vi "Finish.vi"   [LabVIEW 2019]
doc: "This VI is called just before exiting. It is expected to close I/O refnum, save collected data, etc."
uses:
  refnums.vi
  <vilib>/Rock Robotics/WPI/Utilities/WPI_GetSetVariantRefNum.vi
types:
  T1 = typedef "WPI_MotorControlDeviceRef.ctl" = cluster{"DeviceStatus":errorcluster, "Type":T2, "PWM":cluster{"PWM Channel":T3, "DeadBand":T4}, "CAN":cluster{"Device Number":u8, "SetOutput VI Ref":variant, "GetOutput VI Ref":variant, "Enable VI Ref":variant, "Disable VI Ref":variant, "Data":variant}, "Invert":bool, "DIO PWM":cluster{"PWM \"Enable\" Channel":T3, "DIOChannel":T5, "PWM Rate":dbl}}
  T2 = typedef "WPI_MotorControlType.ctl" = enum16{"PWM", "CAN", "DIO PWM"}
  T3 = typedef "FPGA_DIOPWMChannel.ctl" = enum8{"PWM 0", "PWM 1", "PWM 2", "PWM 3", "PWM 4", "PWM 5", "PWM 6", "PWM 7", "PWM 8", "PWM 9", "PWM MXP 0", "PWM MXP 1", "PWM MXP 2", "PWM MXP 3", "PWM MXP 4", "PWM MXP 5", "PWM MXP 6", "PWM MXP 7", "PWM MXP 8", "PWM MXP 9", "Invalid"}
  T4 = typedef "WPI_PWMDeadband.ctl" = cluster{"Name":string, "maxPositivePwm":i32, "minPositivePwm":i32, "centerPwm":i32, "maxNegativePwm":i32, "minNegativePwm":i32, "angularRange":u16}
  T5 = typedef "FPGA_DIOChannel.ctl" = enum8{"DIO 0", "DIO 1", "DIO 2", "DIO 3", "DIO 4", "DIO 5", "DIO 6", "DIO 7", "DIO 8", "DIO 9", "DIO MXP 0", "DIO MXP 1", "DIO MXP 2", "DIO MXP 3", "DIO MXP 4", "DIO MXP 5", "DIO MXP 6", "DIO MXP 7", "DIO MXP 8", "DIO MXP 9", "DIO MXP 10", "DIO MXP 11", "DIO MXP 12", "DIO MXP 13", "DIO MXP 14", "DIO MXP 15", "SPI Port CS1", "SPI Port CS2", "SPI Port CS3", "SPI Port MISO", "SPI Port MOSI", "Invalid"}
  T6 = typedef "WPI_PotentiometerDevRef.ctl" = cluster{"DevStatus":errorcluster, "Analog Channel":T7, "Invert Output":bool}
  T7 = typedef "FPGA_AIChannel.ctl" = enum8{"AI 0", "AI 1", "AI 2", "AI 3", "AI MXP 0", "AI MXP 1", "AI MXP 2", "AI MXP 3", "Invalid"}
  T8 = typedef "WPI_AnalogChannelDevRef.ctl" = cluster{"DevStatus":errorcluster, "Analog Channel":T7}
  T9 = typedef "WPI_SolenoidDevRef.ctl" = cluster{"DevStatus":errorcluster, "Pneumatics Control Module":u8, "Forward Solenoid Channel":T10, "Reverse Solenoid Channel":T10}
  T10 = typedef "WPI_SolenoidChannel.ctl" = enum8{"Solenoid 0", "Solenoid 1", "Solenoid 2", "Solenoid 3", "Solenoid 4", "Solenoid 5", "Solenoid 6", "Solenoid 7", "Invalid"}
  T11 = typedef "WPI_SwitchDevRef.ctl" = cluster{"DevStatus":errorcluster, "DIO Channel":T5, "CntIndex":T12, "Normally Closed":bool}
  T12 = typedef "FPGA_CounterCtrSystemIndex.ctl" = enum8{"Ctr 0", "Ctr 1", "Ctr 2", "Ctr 3", "Ctr 4", "Ctr 5", "Ctr 6", "Ctr 7", "Invalid"}
  T13 = typedef "WPI_CounterDevRef.ctl" = cluster{"DevStatus":errorcluster, "CntIndex":T12}
  T14 = typedef "WPI_JoystickDevRef.ctl" = cluster{"Device":T15}
  T15 = typedef "WPI_JoystickDeviceEnum.ctl" = enum16{"USB 0", "USB 1", "USB 2", "USB 3", "USB 4", "USB 5"}
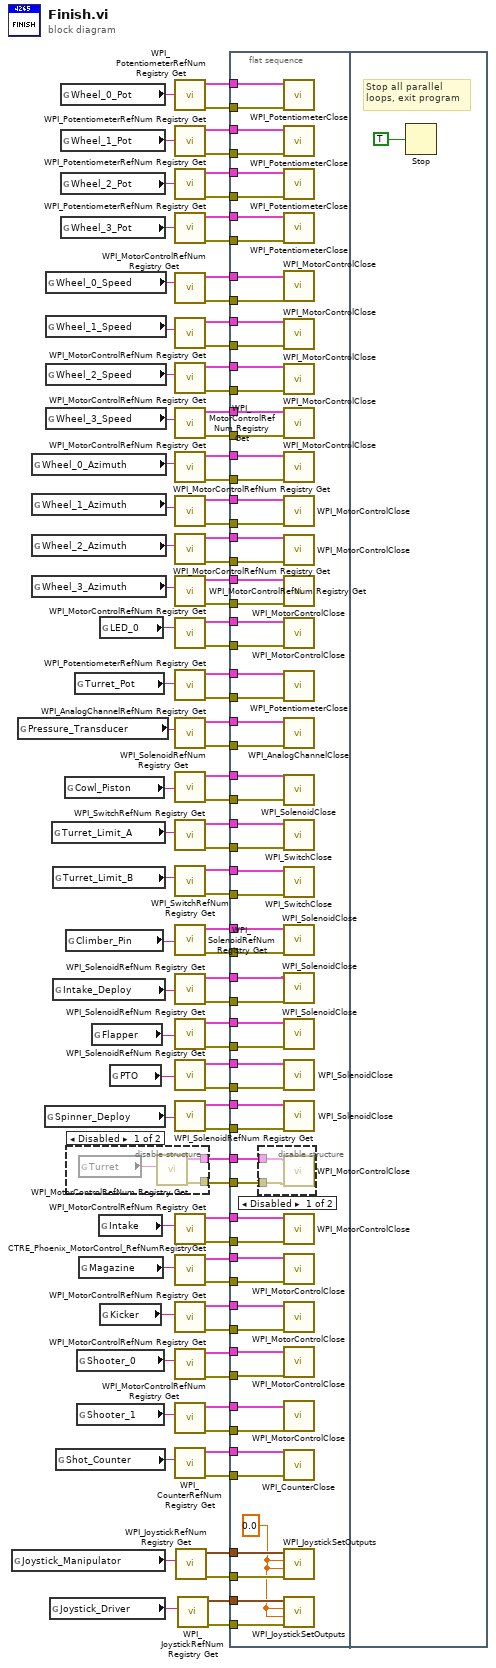
[diagram p0: block diagram]
diagram:
  n1 = global read "refnums.vi" "Joystick_Manipulator"() -> (w6:string)
  n2 = global read "refnums.vi" "Pressure_Transducer"() -> (w56:string)
  n3 = global read "refnums.vi" "Wheel_0_Azimuth"() -> (w83:string)
  n4 = global read "refnums.vi" "Wheel_1_Azimuth"() -> (w82:string)
  n5 = global read "refnums.vi" "Wheel_2_Azimuth"() -> (w81:string)
  n6 = global read "refnums.vi" "Wheel_3_Azimuth"() -> (w80:string)
  n7 = global read "refnums.vi" "Spinner_Deploy"() -> (w21:string)
  n8 = global read "refnums.vi" "Wheel_0_Speed"() -> (w87:string)
  n9 = global read "refnums.vi" "Wheel_1_Speed"() -> (w86:string)
  n10 = global read "refnums.vi" "Wheel_2_Speed"() -> (w85:string)
  n11 = global read "refnums.vi" "Wheel_3_Speed"() -> (w84:string)
  n12 = global read "refnums.vi" "Joystick_Driver"() -> (w1:string)
  n13 = global read "refnums.vi" "Turret_Limit_A"() -> (w11:string)
  n14 = global read "refnums.vi" "Turret_Limit_B"() -> (w10:string)
  n15 = global read "refnums.vi" "Intake_Deploy"() -> (w30:string)
  n16 = global read "refnums.vi" "Shot_Counter"() -> (w8:string)
  n17 = global read "refnums.vi" "Wheel_0_Pot"() -> (w95:string)
  n18 = global read "refnums.vi" "Wheel_1_Pot"() -> (w93:string)
  n19 = global read "refnums.vi" "Wheel_2_Pot"() -> (w92:string)
  n20 = global read "refnums.vi" "Wheel_3_Pot"() -> (w91:string)
  n21 = global read "refnums.vi" "Cowl_Piston"() -> (w53:string)
  n22 = global read "refnums.vi" "Climber_Pin"() -> (w33:string)
  n23 = disable-structure shown="Disabled" {
    disable-tunnel: [w97 _] -> w35
    disable-tunnel: [w96 _] -> w34
    frame Disabled {
      n24 = global read "refnums.vi" "Turret"() -> (w98:string)
      n25 = call <vilib>:"WPI_MotorControlRefNum Registry Get.vi"("refnum name"=w98) -> ("error out"=w96:errorcluster, "MotorControlDevRef"=w97:T1)  [unwired: 9 in]
    }
    frame Enabled {
    }
  }
  n26 = global read "refnums.vi" "Turret_Pot"() -> (w18:string)
  n27 = global read "refnums.vi" "Shooter_0"() -> (w45:string)
  n28 = global read "refnums.vi" "Shooter_1"() -> (w44:string)
  n29 = global read "refnums.vi" "Magazine"() -> (w50:string)
  n30 = global read "refnums.vi" "Flapper"() -> (w29:string)
  n31 = global read "refnums.vi" "Intake"() -> (w38:string)
  n32 = global read "refnums.vi" "LED_0"() -> (w71:string)
  n33 = global read "refnums.vi" "Kicker"() -> (w41:string)
  n34 = global read "refnums.vi" "PTO"() -> (w24:string)
  n35 = call <vilib>:"WPI_PotentiometerRefNum Registry Get.vi"("refnum name"=w95) -> ("error out"=w69:errorcluster, "PotDevRef"=w94:T6)  [unwired: 9 in]
  n36 = call <vilib>:"WPI_PotentiometerRefNum Registry Get.vi"("refnum name"=w93) -> ("error out"=w68:errorcluster, "PotDevRef"=w90:T6)  [unwired: 9 in]
  n37 = call <vilib>:"WPI_PotentiometerRefNum Registry Get.vi"("refnum name"=w92) -> ("error out"=w67:errorcluster, "PotDevRef"=w89:T6)  [unwired: 9 in]
  n38 = call <vilib>:"WPI_PotentiometerRefNum Registry Get.vi"("refnum name"=w91) -> ("error out"=w66:errorcluster, "PotDevRef"=w88:T6)  [unwired: 9 in]
  n39 = call <vilib>:"WPI_MotorControlRefNum Registry Get.vi"("refnum name"=w87) -> ("error out"=w65:errorcluster, "MotorControlDevRef"=w79:T1)  [unwired: 9 in]
  n40 = call <vilib>:"WPI_MotorControlRefNum Registry Get.vi"("refnum name"=w86) -> ("error out"=w64:errorcluster, "MotorControlDevRef"=w78:T1)  [unwired: 9 in]
  n41 = call <vilib>:"WPI_MotorControlRefNum Registry Get.vi"("refnum name"=w85) -> ("error out"=w63:errorcluster, "MotorControlDevRef"=w77:T1)  [unwired: 9 in]
  n42 = call <vilib>:"WPI_MotorControlRefNum Registry Get.vi"("refnum name"=w84) -> ("error out"=w62:errorcluster, "MotorControlDevRef"=w76:T1)  [unwired: 9 in]
  n43 = call <vilib>:"WPI_MotorControlRefNum Registry Get.vi"("refnum name"=w83) -> ("error out"=w61:errorcluster, "MotorControlDevRef"=w75:T1)  [unwired: 9 in]
  n44 = call <vilib>:"WPI_MotorControlRefNum Registry Get.vi"("refnum name"=w82) -> ("error out"=w60:errorcluster, "MotorControlDevRef"=w74:T1)  [unwired: 9 in]
  n45 = call <vilib>:"WPI_MotorControlRefNum Registry Get.vi"("refnum name"=w81) -> ("error out"=w59:errorcluster, "MotorControlDevRef"=w73:T1)  [unwired: 9 in]
  n46 = call <vilib>:"WPI_MotorControlRefNum Registry Get.vi"("refnum name"=w80) -> ("error out"=w58:errorcluster, "MotorControlDevRef"=w72:T1)  [unwired: 9 in]
  n47 = call <vilib>:"WPI_MotorControlRefNum Registry Get.vi"("refnum name"=w71) -> ("error out"=w57:errorcluster, "MotorControlDevRef"=w70:T1)  [unwired: 9 in]
  n48 = call <vilib>:"WPI_PotentiometerRefNum Registry Get.vi"("refnum name"=w18) -> ("error out"=w16:errorcluster, "PotDevRef"=w17:T6)  [unwired: 9 in]
  n49 = call <vilib>:"WPI_AnalogChannelRefNum Registry Get.vi"("refnum name"=w56) -> ("error out"=w54:errorcluster, "AIDeviceRef"=w55:T8)  [unwired: 9 in]
  n50 = call <vilib>:"WPI_SolenoidRefNum Registry Get.vi"("refnum name"=w53) -> ("error out"=w51:errorcluster, "SolenoidDevRef"=w52:T9)  [unwired: 9 in]
  n51 = call <vilib>:"WPI_SwitchRefNum Registry Get.vi"("refnum name"=w11) -> ("error out"=w14:errorcluster, "SwitchDevRef"=w15:T11)  [unwired: 9 in]
  n52 = call <vilib>:"WPI_SwitchRefNum Registry Get.vi"("refnum name"=w10) -> ("error out"=w12:errorcluster, "SwitchDevRef"=w13:T11)  [unwired: 9 in]
  n53 = call <vilib>:"WPI_SolenoidRefNum Registry Get.vi"("refnum name"=w33) -> ("error out"=w31:errorcluster, "SolenoidDevRef"=w32:T9)  [unwired: 9 in]
  n54 = call <vilib>:"WPI_SolenoidRefNum Registry Get.vi"("refnum name"=w30) -> ("error out"=w27:errorcluster, "SolenoidDevRef"=w28:T9)  [unwired: 9 in]
  n55 = call <vilib>:"WPI_SolenoidRefNum Registry Get.vi"("refnum name"=w29) -> ("error out"=w25:errorcluster, "SolenoidDevRef"=w26:T9)  [unwired: 9 in]
  n56 = call <vilib>:"WPI_SolenoidRefNum Registry Get.vi"("refnum name"=w24) -> ("error out"=w22:errorcluster, "SolenoidDevRef"=w23:T9)  [unwired: 9 in]
  n57 = call <vilib>:"WPI_SolenoidRefNum Registry Get.vi"("refnum name"=w21) -> ("error out"=w19:errorcluster, "SolenoidDevRef"=w20:T9)  [unwired: 9 in]
  n58 = call <vilib>:"WPI_MotorControlRefNum Registry Get.vi"("refnum name"=w38) -> ("error out"=w36:errorcluster, "MotorControlDevRef"=w37:T1)  [unwired: 9 in]
  n59 = call <vilib>:"CTRE_Phoenix_MotorControl_RefNumRegistryGet.vi"("refnum name"=w50) -> ("error out"=w48:errorcluster, "PhoenixMotorControlDevRef"=w49:T1)  [unwired: 9 in]
  n60 = call <vilib>:"WPI_MotorControlRefNum Registry Get.vi"("refnum name"=w41) -> ("error out"=w39:errorcluster, "MotorControlDevRef"=w40:T1)  [unwired: 9 in]
  n61 = call <vilib>:"WPI_MotorControlRefNum Registry Get.vi"("refnum name"=w45) -> ("error out"=w46:errorcluster, "MotorControlDevRef"=w47:T1)  [unwired: 9 in]
  n62 = call <vilib>:"WPI_MotorControlRefNum Registry Get.vi"("refnum name"=w44) -> ("error out"=w42:errorcluster, "MotorControlDevRef"=w43:T1)  [unwired: 9 in]
  n63 = call <vilib>:"WPI_CounterRefNum Registry Get.vi"("refnum name"=w8) -> ("error out"=w7:errorcluster, "CounterDevRef"=w9:T13)  [unwired: 9 in]
  n64 = call <vilib>:"WPI_JoystickRefNum Registry Get.vi"("refnum name"=w6) -> ("error out"=w4:errorcluster, "JoystickDevRef"=w5:T14)  [unwired: 9 in]
  n65 = call <vilib>:"WPI_JoystickRefNum Registry Get.vi"("refnum name"=w1) -> ("error out"=w2:errorcluster, "JoystickDevRef"=w3:T14)  [unwired: 9 in]
  n66 = flat-sequence {
    tunnel: w94 -> [w163]
    tunnel: w90 -> [w162]
    tunnel: w89 -> [w161]
    tunnel: w88 -> [w160]
    tunnel: w79 -> [w159]
    tunnel: w78 -> [w158]
    tunnel: w77 -> [w157]
    tunnel: w76 -> [w156]
    tunnel: w75 -> [w155]
    tunnel: w74 -> [w154]
    tunnel: w73 -> [w153]
    tunnel: w72 -> [w152]
    tunnel: w70 -> [w151]
    tunnel: w69 -> [w150]
    tunnel: w68 -> [w149]
    tunnel: w67 -> [w148]
    tunnel: w66 -> [w147]
    tunnel: w65 -> [w146]
    tunnel: w64 -> [w145]
    tunnel: w63 -> [w144]
    tunnel: w62 -> [w143]
    tunnel: w61 -> [w142]
    tunnel: w60 -> [w141]
    tunnel: w59 -> [w140]
    tunnel: w58 -> [w139]
    tunnel: w57 -> [w138]
    tunnel: w55 -> [w137]
    tunnel: w54 -> [w136]
    tunnel: w52 -> [w135]
    tunnel: w51 -> [w134]
    tunnel: w47 -> [w133]
    tunnel: w46 -> [w132]
    tunnel: w49 -> [w131]
    tunnel: w48 -> [w130]
    tunnel: w43 -> [w129]
    tunnel: w42 -> [w128]
    tunnel: w40 -> [w127]
    tunnel: w39 -> [w126]
    tunnel: w37 -> [w125]
    tunnel: w36 -> [w124]
    tunnel: w35 -> [w123]
    tunnel: w34 -> [w122]
    tunnel: w32 -> [w121]
    tunnel: w31 -> [w120]
    tunnel: w28 -> [w119]
    tunnel: w27 -> [w118]
    tunnel: w26 -> [w117]
    tunnel: w25 -> [w116]
    tunnel: w23 -> [w115]
    tunnel: w22 -> [w114]
    tunnel: w20 -> [w113]
    tunnel: w19 -> [w112]
    tunnel: w17 -> [w111]
    tunnel: w16 -> [w110]
    tunnel: w15 -> [w109]
    tunnel: w13 -> [w108]
    tunnel: w12 -> [w107]
    tunnel: w14 -> [w106]
    tunnel: w9 -> [w105]
    tunnel: w7 -> [w104]
    tunnel: w5 -> [w103]
    tunnel: w4 -> [w102]
    tunnel: w3 -> [w101]
    tunnel: w2 -> [w100]
    frame #0 {
      w99 = sgl 0.0 ("Left Rumble")
      n67 = disable-structure shown="Disabled" {
        disable-tunnel: w123 -> [w165 _]
        disable-tunnel: w122 -> [w164 _]
        frame Disabled {
          n68 = call <vilib>:"WPI_MotorControlClose.vi"("error in"=w164, "MotorControlDevRef"=w165) -> ()  [unwired: 9 in, 1 out]
        }
        frame Enabled {
        }
      }
      n69 = call <vilib>:"WPI_PotentiometerClose.vi"("error in"=w150, "PotDevRef"=w163) -> ()  [unwired: 9 in, 1 out]
      n70 = call <vilib>:"WPI_PotentiometerClose.vi"("error in"=w149, "PotDevRef"=w162) -> ()  [unwired: 9 in, 1 out]
      n71 = call <vilib>:"WPI_PotentiometerClose.vi"("error in"=w148, "PotDevRef"=w161) -> ()  [unwired: 9 in, 1 out]
      n72 = call <vilib>:"WPI_PotentiometerClose.vi"("error in"=w147, "PotDevRef"=w160) -> ()  [unwired: 9 in, 1 out]
      n73 = call <vilib>:"WPI_MotorControlClose.vi"("error in"=w146, "MotorControlDevRef"=w159) -> ()  [unwired: 9 in, 1 out]
      n74 = call <vilib>:"WPI_MotorControlClose.vi"("error in"=w145, "MotorControlDevRef"=w158) -> ()  [unwired: 9 in, 1 out]
      n75 = call <vilib>:"WPI_MotorControlClose.vi"("error in"=w144, "MotorControlDevRef"=w157) -> ()  [unwired: 9 in, 1 out]
      n76 = call <vilib>:"WPI_MotorControlClose.vi"("error in"=w143, "MotorControlDevRef"=w156) -> ()  [unwired: 9 in, 1 out]
      n77 = call <vilib>:"WPI_MotorControlClose.vi"("error in"=w142, "MotorControlDevRef"=w155) -> ()  [unwired: 9 in, 1 out]
      n78 = call <vilib>:"WPI_MotorControlClose.vi"("error in"=w141, "MotorControlDevRef"=w154) -> ()  [unwired: 9 in, 1 out]
      n79 = call <vilib>:"WPI_MotorControlClose.vi"("error in"=w140, "MotorControlDevRef"=w153) -> ()  [unwired: 9 in, 1 out]
      n80 = call <vilib>:"WPI_MotorControlClose.vi"("error in"=w139, "MotorControlDevRef"=w152) -> ()  [unwired: 9 in, 1 out]
      n81 = call <vilib>:"WPI_MotorControlClose.vi"("error in"=w138, "MotorControlDevRef"=w151) -> ()  [unwired: 9 in, 1 out]
      n82 = call <vilib>:"WPI_PotentiometerClose.vi"("error in"=w110, "PotDevRef"=w111) -> ()  [unwired: 9 in, 1 out]
      n83 = call <vilib>:"WPI_AnalogChannelClose.vi"("error in (no error)"=w136, "AIDeviceRef"=w137) -> ()  [unwired: 9 in, 1 out]
      n84 = call <vilib>:"WPI_SolenoidClose.vi"("error in (no error)"=w134, "SolenoidDevRef"=w135) -> ()  [unwired: 9 in, 1 out]
      n85 = call <vilib>:"WPI_SwitchClose.vi"("error in (no error)"=w106, "SwitchDevRef"=w109) -> ()  [unwired: 9 in, 1 out]
      n86 = call <vilib>:"WPI_SwitchClose.vi"("error in (no error)"=w107, "SwitchDevRef"=w108) -> ()  [unwired: 9 in, 1 out]
      n87 = call <vilib>:"WPI_SolenoidClose.vi"("error in (no error)"=w120, "SolenoidDevRef"=w121) -> ()  [unwired: 9 in, 1 out]
      n88 = call <vilib>:"WPI_SolenoidClose.vi"("error in (no error)"=w118, "SolenoidDevRef"=w119) -> ()  [unwired: 9 in, 1 out]
      n89 = call <vilib>:"WPI_SolenoidClose.vi"("error in (no error)"=w116, "SolenoidDevRef"=w117) -> ()  [unwired: 9 in, 1 out]
      n90 = call <vilib>:"WPI_SolenoidClose.vi"("error in (no error)"=w114, "SolenoidDevRef"=w115) -> ()  [unwired: 9 in, 1 out]
      n91 = call <vilib>:"WPI_SolenoidClose.vi"("error in (no error)"=w112, "SolenoidDevRef"=w113) -> ()  [unwired: 9 in, 1 out]
      n92 = call <vilib>:"WPI_MotorControlClose.vi"("error in"=w124, "MotorControlDevRef"=w125) -> ()  [unwired: 9 in, 1 out]
      n93 = call <vilib>:"WPI_MotorControlClose.vi"("error in"=w130, "MotorControlDevRef"=w131) -> ()  [unwired: 9 in, 1 out]
      n94 = call <vilib>:"WPI_MotorControlClose.vi"("error in"=w126, "MotorControlDevRef"=w127) -> ()  [unwired: 9 in, 1 out]
      n95 = call <vilib>:"WPI_MotorControlClose.vi"("error in"=w132, "MotorControlDevRef"=w133) -> ()  [unwired: 9 in, 1 out]
      n96 = call <vilib>:"WPI_MotorControlClose.vi"("error in"=w128, "MotorControlDevRef"=w129) -> ()  [unwired: 9 in, 1 out]
      n97 = call <vilib>:"WPI_CounterClose.vi"("error in (no error)"=w104, "CounterDevRef"=w105) -> ()  [unwired: 9 in, 1 out]
      n98 = call <vilib>:"WPI_JoystickSetOutputs.vi"("error in (no error)"=w102, "Right Rumble"=w99, "Left Rumble"=w99, "JoystickDevRef"=w103) -> ()  [unwired: 6 in, 2 out]
      n99 = call <vilib>:"WPI_JoystickSetOutputs.vi"("error in (no error)"=w100, "Right Rumble"=w99, "Left Rumble"=w99, "JoystickDevRef"=w101) -> ()  [unwired: 6 in, 2 out]
    }
    frame #1 {
      # "Stop all parallel\nloops, exit program"
      n100 = Stop(stop? (T)=TRUE ("Quit")) -> ()
    }
  }
